vi "Set Core Transfer Settings.vi"(8 "error in (no error)":errorcluster, 10 "transfer configuration":T1={"name"="Transfer"}, 11 "Item Ref in":T2 format="%.0x") -> (0 "error out":errorcluster, 3 "Item Ref out":T2 format="%.0x")   [LabVIEW 2017, in "DSF System Explorer.lvlib"]
uses:
  DSF System Explorer.lvlib
  <vilib>/NI Veristand/Custom Device API/Custom Device Item Ref.ctl
  DSF Core.lvlibp/Typedefs/Core Transfer Configuration.ctl
  <vilib>/NI Veristand/Custom Device API/Set Item Property (Variant).vi
  <vilib>/NI Veristand/Custom Device API/Custom Device API.lvlib
  DSF Core.lvlibp/Classes/Configuration/Base/Transfer/Transfer Configuration.lvclass
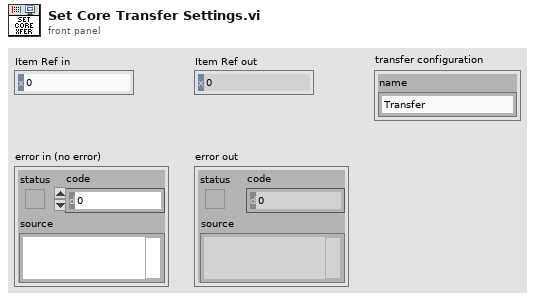
[diagram p1: front panel]
types:
  T1 = typedef "DSF Core.lvlibp/Transfer Configuration.lvclass/Core Transfer Configuration.ctl" = cluster{"name":string}
  T2 = typedef "Custom Device API.lvlib/Custom Device Item Ref.ctl" = u64
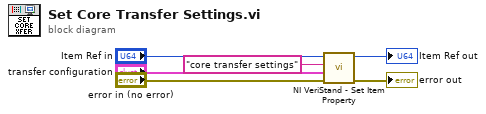
[diagram p0: block diagram]
diagram:
  n1 = call-poly <vilib>:"NI VeriStand - Set Item Property.vi"("error in (no error)"="error in (no error)", "Value"="transfer configuration", "Property Name"="core transfer settings" ("dsf options"), "Item Ref in"="Item Ref in") -> ("error out"=→"error out":errorcluster, "Item Ref out"=→"Item Ref out":T2)  [unwired: 5 in, 1 out]
